vi "Self-Test.vi"(8 "error in (no error)":errorcluster, 11 "34401 in":refnum<class "34401.lvclass">) -> (0 "error out":errorcluster, 1 "Self-Test Message":string, 2 "Self-Test Result (Pass=T)":bool, 3 "34401 out":refnum<class "34401.lvclass">)   [LabVIEW 2018, in "34401.lvlib" / "34401.lvclass"]
uses:
  34401.lvclass
  34401.lvclass/34401.ctl
  <instrlib>/Agilent 34401/Agilent 34401.lvlib
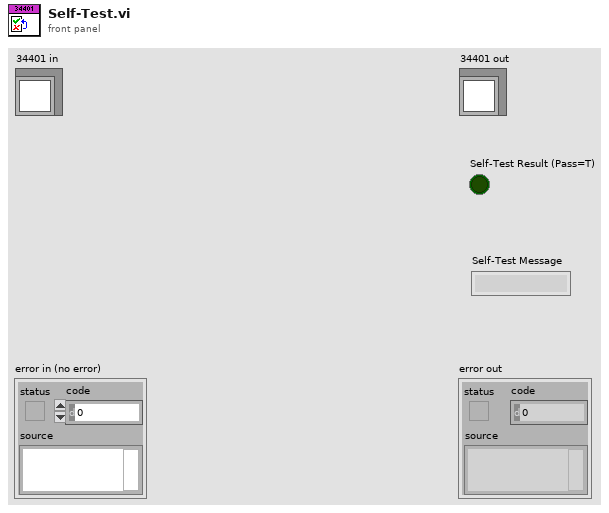
[diagram p1: front panel]
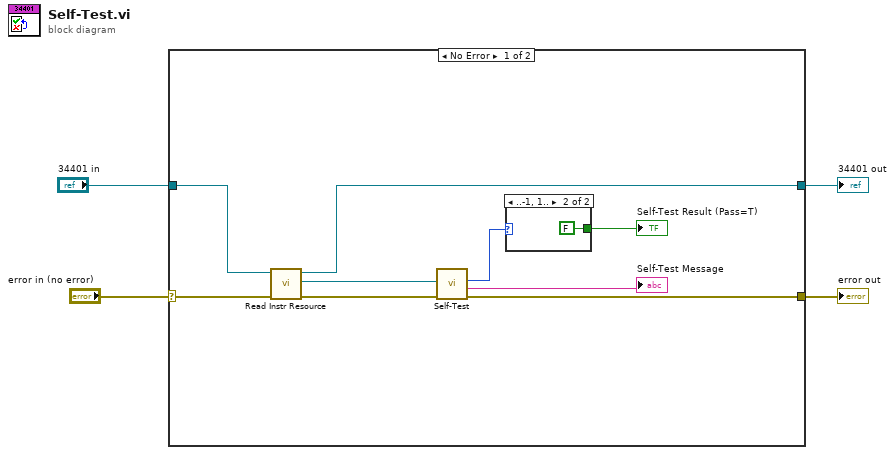
[diagram p0: block diagram]
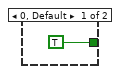
[diagram p2: hidden frame]
diagram:
  n1 = case shown="No Error" "error in (no error)" {
    selector: "error in (no error)" -> [w13 w16]
    tunnel: "34401 in" -> [w12 w17]
    tunnel: [w9 w17] -> w2
    tunnel: [w8 w16] -> w1
    frame No Error {
      n2 = call "Read Instr Resource.vi"("error in (no error)"=w13, "34401 in"=w12) -> ("error out"=w11:errorcluster, "Instr Resource"=w10:refnum<visa-resource-name>, "34401 out"=w9:refnum<class "34401.lvclass">)  [unwired: 7 in]
      n3 = call <instrlib>:"Self-Test.vi"("error in (no error)"=w11, "VISA resource name"=w10) -> ("error out"=w8:errorcluster, "Self-Test Result Message"=→"Self-Test Message":string, "Self-Test Result Code"=w7:i32)  [unwired: 6 in, 1 out]
      n4 = case shown="..-1, 1.." w7 {
        tunnel: [TRUE FALSE] -> w6
        frame 0, Default {
        }
        frame ..-1, 1.. {
        }
      }
      "Self-Test Result (Pass=T)" <- w6
    }
    frame Error {
    }
  }
  "error out" <- w1
  "34401 out" <- w2
